vi "Start.vi"(8 "error in (no error)":errorcluster, 10 "Sequence Name":string, 11 "Sequencing in":refnum<class "Sequencing.lvclass">) -> (0 "error out":errorcluster, 3 "Sequencing out":refnum<class "Sequencing.lvclass">)   [LabVIEW 2020, in "VolatusSeq.lvlib" / "Sequencing.lvclass"]
uses:
  Sequencing.lvclass
  Sequencing.lvclass/Sequencing.ctl
  Sequence/Sequence.lvclass
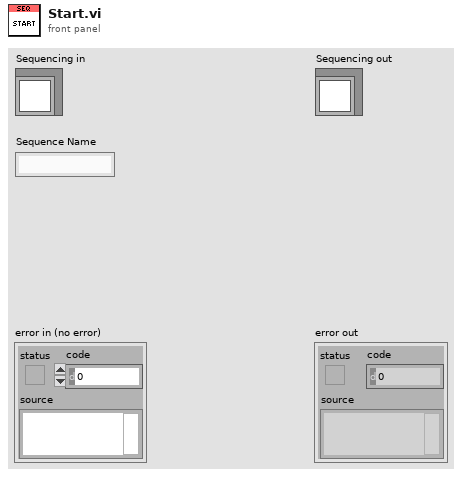
[diagram p1: front panel]
types:
  T1 = typedef "VolatusSeq.lvlib/Sequence Status.ctl" = cluster{"Name":string, "State":string, "Time":T2, "Running":bool}
  T2 = typedef "VolatusSeq.lvlib/Sequence Time.ctl" = cluster{"Abort":bool, "Seq Time":dbl, "State Time":dbl, "Wall Time":dbl}
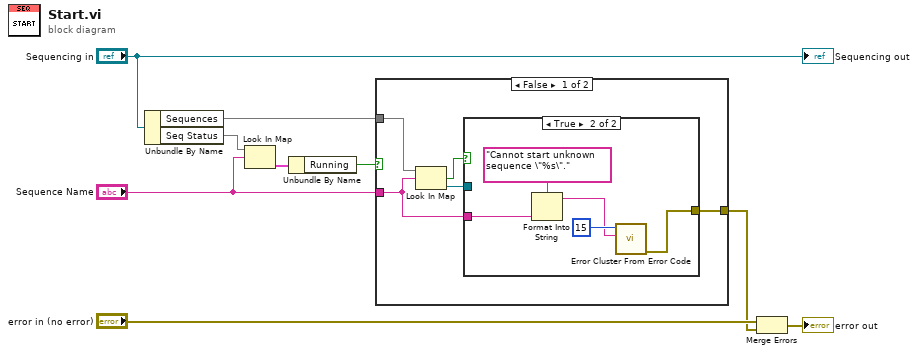
[diagram p0: block diagram]
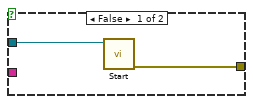
[diagram p2: hidden frame]
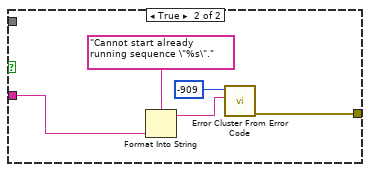
[diagram p3: hidden frame]
diagram:
  n1 = Unbundle By Name("Sequencing in") -> ("Sequences"=w2:map{string, refnum<class "Sequence.lvclass">}, "Seq Status"=w6:map{string, T1})
  n2 = Look In Map(map=w6, key="Sequence Name") -> (value=w5:T1)  [unwired: 1 in, 1 out]
  n3 = Unbundle By Name(w5) -> ("Running"=w1:bool)
  n4 = case shown="False" w1 {
    tunnel: [w13 w23] -> w7
    tunnel: "Sequence Name" -> [w11 w22]
    tunnel: w2 -> [w10 _]
    frame False {
      n5 = Look In Map(map=w10, key=w11) -> (key not found?=w12:bool, value=w14:refnum<class "Sequence.lvclass">)  [unwired: 1 in]
      n6 = case shown="True" w12 {
        tunnel: w14 -> [w16 _]
        tunnel: [w15 w17] -> w13
        tunnel: w11 -> [_ w20]
        frame False {
          n7 = call "Start.vi"("Sequence in"=w16) -> ("error out"=w15:errorcluster)  [unwired: 9 in, 1 out]
        }
        frame True {
          n8 = Format Into String(format string="Cannot start unknown sequence \"%s\".", w20) -> (resulting string=w18:string)  [unwired: 2 in, 1 out]
          n9 = call <vilib>:"Error Cluster From Error Code.vi"("error message (\"\")"=w18, "error code (0)"=15) -> ("error out"=w17:errorcluster)  [unwired: 7 in]
        }
      }
    }
    frame True {
      n10 = Format Into String(format string="Cannot start already running sequence \"%s\".", w22) -> (resulting string=w24:string)  [unwired: 2 in, 1 out]
      n11 = call <vilib>:"Error Cluster From Error Code.vi"("error message (\"\")"=w24, "error code (0)"=-909) -> ("error out"=w23:errorcluster)  [unwired: 7 in]
    }
  }
  n12 = Merge Errors("error in (no error)", w7) -> (→"error out":errorcluster)
  "Sequencing out" <- "Sequencing in"
